vi "ResonanceAnalyzer.vi"() -> ()   [LabVIEW 2014]
uses:
  <vilib>/Utility/file.llb/Read From Spreadsheet File (DBL).vi
panel:
  in  "?":enum32{"Simulation", "Experiment"}(tab)
  in  "Input Parameters":T1
  in  "file path (dialog if empty)":path
  out "Results":T2
  out "Resonance Curve":cluster{"all rows":dbl[], "all rows":dbl[]}(graph)
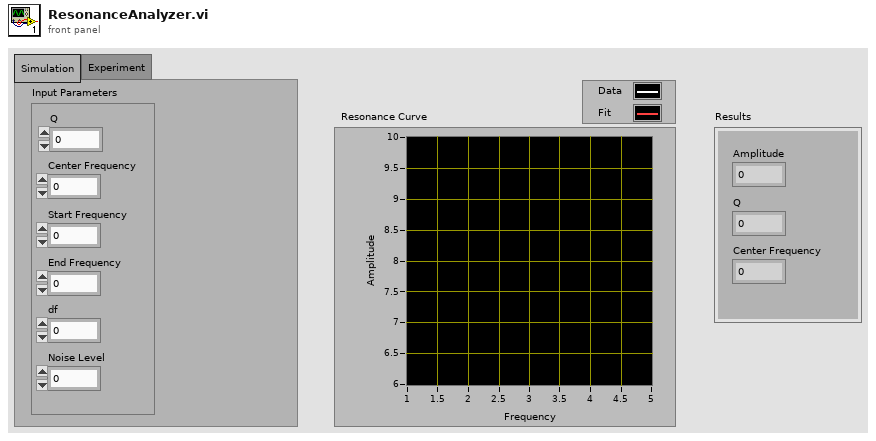
[diagram p1: front panel]
types:
  T1 = cluster{"Q":dbl, "Center Frequency":dbl, "Start Frequency":dbl, "End Frequency":dbl, "df":dbl, "Noise Level":dbl}
  T2 = cluster{"Amplitude":dbl, "Q":dbl, "Center Frequency":dbl}
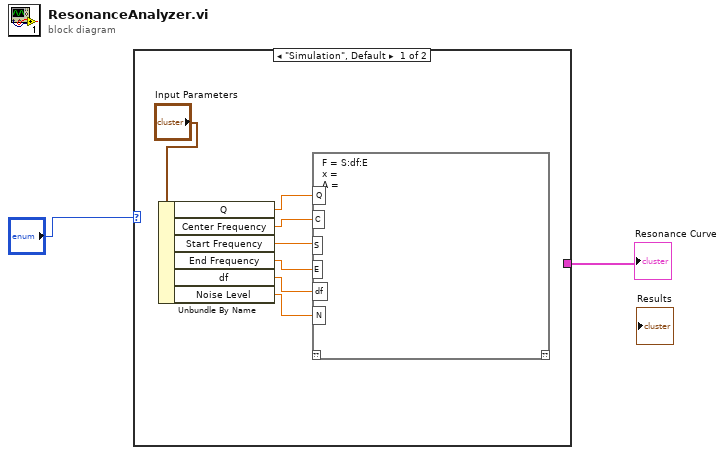
[diagram p0: block diagram]
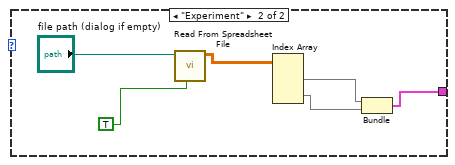
[diagram p2: hidden frame]
diagram:
  n1 = case shown="\"Simulation\", Default" "?" {
    tunnel: [_ w11] -> w2
    frame "Simulation", Default {
      n2 = Unbundle By Name("Input Parameters") -> ("Q"=w8:dbl, "Center Frequency"=w7:dbl, "Start Frequency"=w6:dbl, "End Frequency"=w5:dbl, "df"=w4:dbl, "Noise Level"=w3:dbl)
      n3 = mathscript code="F = S:df:E\nx = \nA ="("S"=w6, "Q"=w8, "C"=w7, "E"=w5, "df"=w4, "N"=w3) -> ()  [unwired: 1 in, 1 out]
    }
    frame "Experiment" {
      n4 = call-poly <vilib>:"Read From Spreadsheet File.vi"("transpose (no:F)"=TRUE, "file path (dialog if empty)"="file path (dialog if empty)") -> ("all rows"=w13:dbl[][])  [unwired: 5 in, 4 out]
      n5 = Index Array(array=w13) -> (element #1=w15:dbl[], element #2=w14:dbl[])  [unwired: 4 in]
      n6 = Bundle("all rows"=w15, "all rows"=w14) -> (w11:cluster{"all rows":dbl[], "all rows":dbl[]})  [unwired: 1 in]
    }
  }
  "Resonance Curve" <- w2
